vi "Merge Data.vi"(8 "error in":errorcluster, 10 "Analyzed":refnum<class "Instrument.lvclass">, 11 "Acquired":refnum<class "Open Path CRD.lvclass">) -> (0 "error out":errorcluster, 3 "tCRD out":refnum<class "Open Path CRD.lvclass">)   [LabVIEW 2015, in "Open Path CRD.lvclass"]
doc: "The VI Merge Data is used strictly here to merge the serial data with the rest of the data. THIS VI WILL BE NO LONGER NECESSARY WHEN ISSUES RELATING TO RT EXE ARE FIXED!!"
uses:
  Open Path CRD.lvclass
  Reusable/Instrument/Instrument.lvclass
  Open Path CRD.lvclass/Open Path CRD.ctl
  Reusable/CRDS/Main/CRDS.lvclass
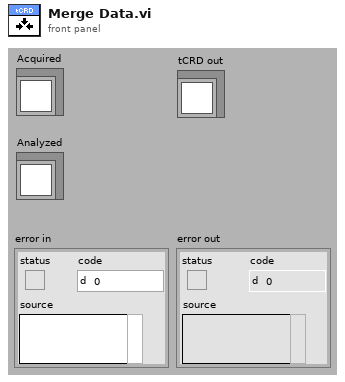
[diagram p1: front panel]
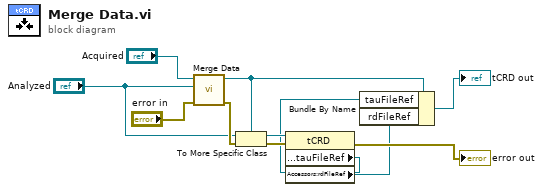
[diagram p0: block diagram]
diagram:
  n1 = call-parent "Merge Data.vi"("error in"="error in", "Analyzed"="Analyzed", "Acquired"="Acquired") -> ("error out"=w10:errorcluster, "CRDS out"=w7:refnum<class "Open Path CRD.lvclass">)  [unwired: 7 in]
  n2 = To More Specific Class(target class=w7, reference="Analyzed", error in=w10) -> (specific class reference=w5:refnum<class "Open Path CRD.lvclass">, error out=w4:errorcluster)
  n3 = property class="tCRD"(reference=w5, error in=w4) -> (error out=→"error out":errorcluster, "Accessors:tauFileRef"=w3:refnum<file>, "Accessors:rdFileRef"=w1:refnum<file>)  [unwired: 1 out]
  n4 = Bundle By Name(cluster=w7, "tauFileRef"=w3, "rdFileRef"=w1) -> (→"tCRD out":refnum<class "Open Path CRD.lvclass">)
